vi "ConvertMeasureData.vi"(9 "select_out_graph":T1, 10 "select_graph":enum8{"TriggerCount", "PulseCount"}(ring), 11 "measurementData":T2[](array[typedef]) {"outMeasurementData"."judgeResult" items=["HI"=1, "GO"=2, "LO"=4]}) -> (2 "Log out":dbl[][](array[numeric]), 3 "Data out":T6(array[cluster]))   [LabVIEW 2020]
uses:
  Public/clusters/CL3IF_MEASUREMENT_DATA.ctl
  Public/clusters/CL3IF_OUTMEASUREMENT_DATA.ctl
  Public/enums/CL3IF_VALUE_INFO.ctl
  Public/enums/CL3IF_JUDGE_RESULT.ctl
  ctrl/select_out.ctl
  Keyence CL-3000.lvlib
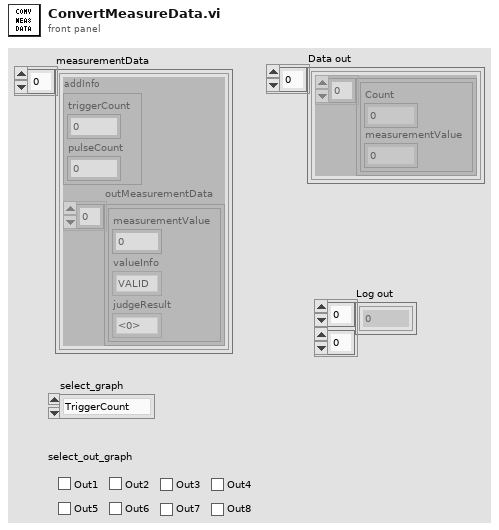
[diagram p1: front panel]
types:
  T1 = typedef "select_out.ctl" = cluster{"out1":bool, "out2":bool, "out3":bool, "out4":bool, "out5":bool, "out6":bool, "out7":bool, "out8":bool}
  T2 = typedef "Keyence CL-3000.lvlib/CL3IF_MEASUREMENT_DATA.ctl" = cluster{"addInfo":cluster{"triggerCount":u32, "pulseCount":i32}, "outMeasurementData":T3[]}
  T3 = typedef "Keyence CL-3000.lvlib/CL3IF_OUTMEASUREMENT_DATA.ctl" = cluster{"measurementValue":i32, "valueInfo":T4, "judgeResult":T5}
  T4 = typedef "Keyence CL-3000.lvlib/CL3IF_VALUE_INFO.ctl" = enum8{"VALID", "JUDGMENTSTANDBY", "INVALID", "OVERDISPRANGE_P", "OVERDISPRANGE_N"}
  T5 = typedef "Keyence CL-3000.lvlib/CL3IF_JUDGE_RESULT.ctl" = u8
  T6 = cluster{cluster{"Count":dbl, "measurementValue":dbl}[]}[]
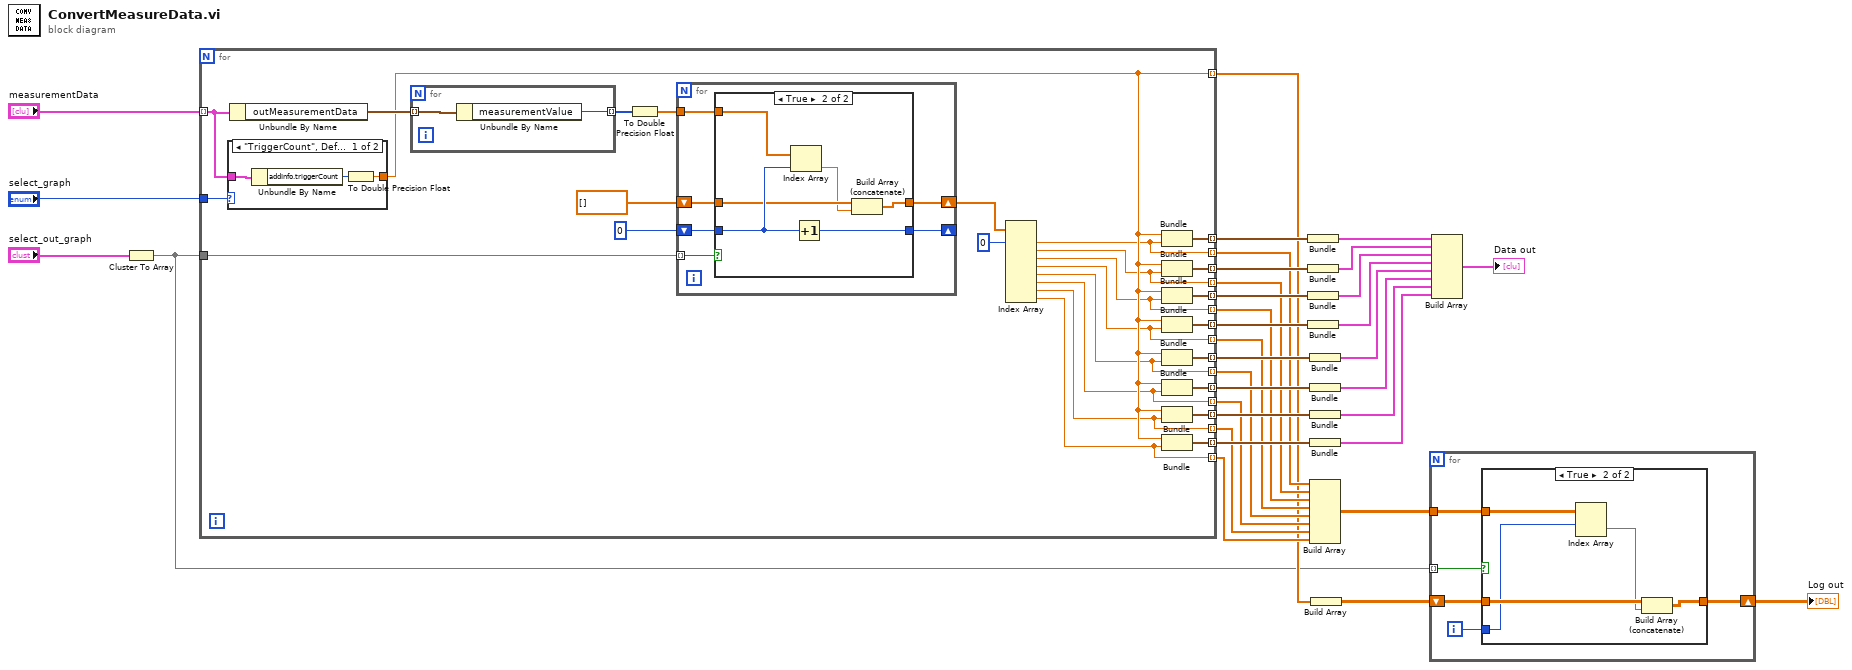
[diagram p0: block diagram]
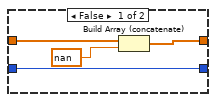
[diagram p3: hidden frame]
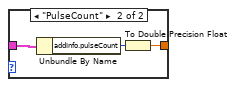
[diagram p4: hidden frame]
diagram:
  n1 = Cluster To Array(cluster="select_out_graph") -> (array=w1:bool[])
  n2 = for {
    tunnel: "measurementData" -> [w60] mode=indexing
    tunnel: [w58] -> w30 mode=indexing
    tunnel: [w56] -> w31 mode=indexing
    tunnel: "select_graph" -> [w55]
    tunnel: [w53] -> w26 mode=indexing
    tunnel: [w52] -> w24 mode=indexing
    tunnel: [w51] -> w22 mode=indexing
    tunnel: [w50] -> w21 mode=indexing
    tunnel: [w49] -> w20 mode=indexing
    tunnel: [w48] -> w19 mode=indexing
    tunnel: [w47] -> w3 mode=indexing
    tunnel: [w41] -> w14 mode=indexing
    tunnel: [w40] -> w13 mode=indexing
    tunnel: [w39] -> w12 mode=indexing
    tunnel: [w38] -> w11 mode=indexing
    tunnel: [w37] -> w10 mode=indexing
    tunnel: [w36] -> w9 mode=indexing
    tunnel: [w35] -> w8 mode=indexing
    tunnel: [w34] -> w7 mode=indexing
    tunnel: w1 -> [w46]
    n3 = case shown="\"TriggerCount\", Default" w55 {
      tunnel: w60 -> [w79 w82]
      tunnel: [w77 w80] -> w47
      frame "TriggerCount", Default {
        n4 = Unbundle By Name(w79) -> ("addInfo.triggerCount"=w78:u32)
        n5 = To Double Precision Float(number=w78) -> (double precision float=w77:dbl)
      }
      frame "PulseCount" {
        n6 = Unbundle By Name(w82) -> ("addInfo.pulseCount"=w81:i32)
        n7 = To Double Precision Float(number=w81) -> (double precision float=w80:dbl)
      }
    }
    n8 = Unbundle By Name(w60) -> ("outMeasurementData"=w59:T3[])
    n9 = for {
      tunnel: w59 -> [w84] mode=indexing
      tunnel: [w83] -> w57 mode=indexing
      n10 = Unbundle By Name(w84) -> ("measurementValue"=w83:i32)
    }
    n11 = To Double Precision Float(number=w57) -> (double precision float=w45:dbl[])
    n12 = for {
      tunnel: w46 -> [w66] mode=indexing
      tunnel: w45 -> [w65]
      shift-right: [w63] -> _
      shift-left: u8 0 -> [w64]
      shift-right: [w61] -> w42
      shift-left: dbl[] [] -> [w62]
      n13 = case shown="True" w66 {
        tunnel: w65 -> [_ w76]
        tunnel: w64 -> [w70 w75]
        tunnel: [w70 w74] -> w63
        tunnel: w62 -> [w69 w73]
        tunnel: [w67 w71] -> w61
        frame False {
          n14 = Build Array (concatenate)(w69, nan) -> (w67:dbl[])
        }
        frame True {
          n15 = Index Array(array=w76, index=w75) -> (element=w72:dbl)
          n16 = Increment(x=w75) -> (x+1=w74:u8)
          n17 = Build Array (concatenate)(w73, w72) -> (w71:dbl[])
        }
      }
    }
    n18 = Index Array(array=w42, index #1=0 ("Žw•W")) -> (element #1=w41:dbl, element #2=w40:dbl, element #3=w39:dbl, element #4=w38:dbl, element #5=w37:dbl, element #6=w36:dbl, element #7=w35:dbl, element #8=w34:dbl)  [unwired: 7 in]
    n19 = Bundle(w47, w41) -> (w58:cluster{dbl, dbl})  [unwired: 1 in]
    n20 = Bundle(w47, w40) -> (w56:cluster{dbl, dbl})  [unwired: 1 in]
    n21 = Bundle(w47, w39) -> (w53:cluster{dbl, dbl})  [unwired: 1 in]
    n22 = Bundle(w47, w38) -> (w52:cluster{dbl, dbl})  [unwired: 1 in]
    n23 = Bundle(w47, w37) -> (w51:cluster{dbl, dbl})  [unwired: 1 in]
    n24 = Bundle(w47, w36) -> (w50:cluster{dbl, dbl})  [unwired: 1 in]
    n25 = Bundle(w47, w35) -> (w49:cluster{dbl, dbl})  [unwired: 1 in]
    n26 = Bundle(w47, w34) -> (w48:cluster{dbl, dbl})  [unwired: 1 in]
  }
  n27 = Bundle(w30) -> (w32:cluster{cluster{dbl, dbl}[]})  [unwired: 1 in]
  n28 = Bundle(w31) -> (w27:cluster{cluster{dbl, dbl}[]})  [unwired: 1 in]
  n29 = Bundle(w26) -> (w25:cluster{cluster{dbl, dbl}[]})  [unwired: 1 in]
  n30 = Bundle(w24) -> (w23:cluster{cluster{dbl, dbl}[]})  [unwired: 1 in]
  n31 = Bundle(w22) -> (w18:cluster{cluster{dbl, dbl}[]})  [unwired: 1 in]
  n32 = Bundle(w21) -> (w17:cluster{cluster{dbl, dbl}[]})  [unwired: 1 in]
  n33 = Bundle(w20) -> (w16:cluster{cluster{dbl, dbl}[]})  [unwired: 1 in]
  n34 = Bundle(w19) -> (w15:cluster{cluster{dbl, dbl}[]})  [unwired: 1 in]
  n35 = Build Array(w14, w13, w12, w11, w10, w9, w8, w7) -> (w6:dbl[][])
  n36 = Build Array(w3) -> (w4:dbl[][])
  n37 = for {
    tunnel: w1 -> [w89] mode=indexing
    tunnel: w6 -> [w87]
    shift-right: [w85] -> w5
    shift-left: w4 -> [w86]
    i -> [w88]
    n38 = case shown="True" w89 {
      tunnel: w88 -> [_ w91]
      tunnel: w87 -> [_ w95]
      tunnel: w86 -> [w90 w94]
      tunnel: [w90 w92] -> w85
      frame False {
      }
      frame True {
        n39 = Index Array(array=w95, index (row)=w91) -> (element=w93:dbl[])  [unwired: 1 in]
        n40 = Build Array (concatenate)(w94, w93) -> (w92:dbl[][])
      }
    }
  }
  "Log out" <- w5
  n41 = Build Array(w32, w27, w25, w23, w18, w17, w16, w15) -> (→"Data out":cluster{cluster{dbl, dbl}[]}[])
